vi "Initialize From Settings.vi"(8 "error in (no error)":errorcluster, 10 "settings":cluster{"key":string, "value":string}[](array[cluster]), 11 "DSF Buffer Converter Transfer Configuration in":refnum<class "DSF Buffer Converter Transfer Configuration.lvclass">) -> (0 "error out":errorcluster, 3 "DSF Buffer Converter Transfer Configuration out":refnum<class "DSF Buffer Converter Transfer Configuration.lvclass">)   [LabVIEW 2017, in "DSF Core.lvlib" / "DSF Buffer Converter Transfer Configuration.lvclass"]
uses:
  DSF Buffer Converter Transfer Configuration.lvclass
  DSF Buffer Converter Transfer Configuration.lvclass/DSF Buffer Converter Transfer Configuration.ctl
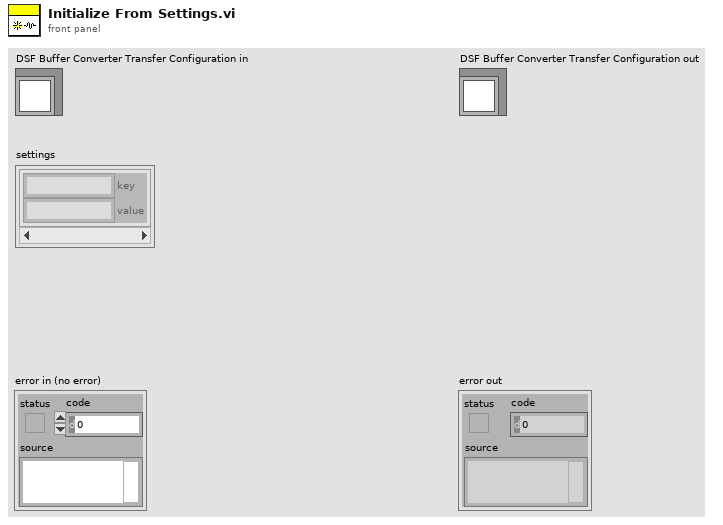
[diagram p1: front panel]
types:
  T1 = cluster{"byte order":enum8{"big-endian", "little-endian"}}
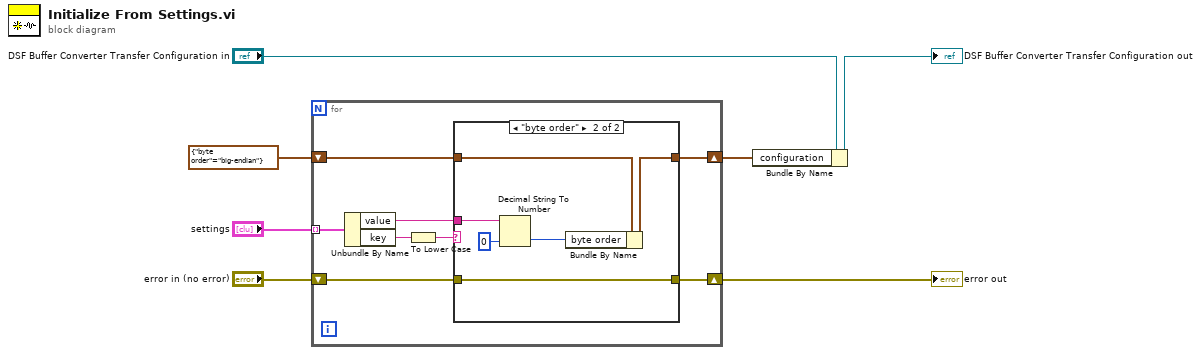
[diagram p0: block diagram]
diagram:
  n1 = for {
    shift-right: [w8] -> w6
    shift-left: "error in (no error)" -> [w14]
    shift-right: [w10] -> w1
    shift-left: T1 {"byte order"=enum."big-endian"} ("configuration") -> [w11]
    tunnel: "settings" -> [w15] mode=indexing
    n2 = Unbundle By Name(w15) -> ("value"=w12:string, "key"=w13:string)
    n3 = To Lower Case(string=w13) -> (all lower case string=w9:string)
    n4 = case shown="\"byte order\"" w9 {
      tunnel: w14 -> [w16 w21]
      tunnel: w12 -> [_ w20]
      tunnel: w11 -> [w17 w23]
      tunnel: [w17 w22] -> w10
      tunnel: [w16 w21] -> w8
      frame Default {
        # "Unknown Setting."
      }
      frame "byte order" {
        n5 = Decimal String To Number(string=w20, default (0L)=u8 0 ("default (0 I32)")) -> (number=w19:u8)  [unwired: 1 in, 1 out]
        n6 = Bundle By Name(cluster=w23, "byte order"=w19) -> (w22:T1)
      }
    }
  }
  "error out" <- w6
  n7 = Bundle By Name(cluster="DSF Buffer Converter Transfer Configuration in", "configuration"=w1) -> (→"DSF Buffer Converter Transfer Configuration out":refnum<class "DSF Buffer Converter Transfer Configuration.lvclass">)
